vi "Calculate Voltage Difference.vi"(0 "Target Value":dbl[](array[numeric]), 2 "PowerUp?":bool, 5 "Start Value":dbl[](array[numeric])) -> (4 "Value  difference":dbl[](array[numeric]))   [LabVIEW 2024, in "devicePowerSequencerCoreLogic.lvlib"]
uses:
  devicePowerSequencerCoreLogic.lvlib
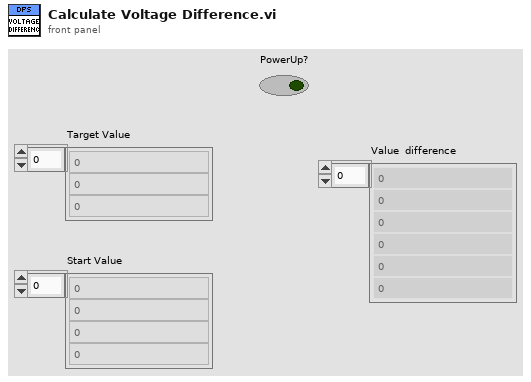
[diagram p1: front panel]
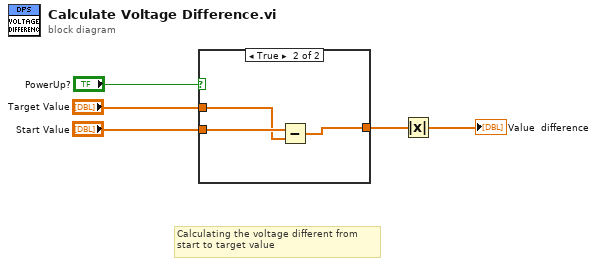
[diagram p0: block diagram]
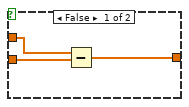
[diagram p2: hidden frame]
diagram:
  # "Calculating the voltage different from \nstart to target value"
  n1 = case shown="True" "PowerUp?" {
    tunnel: "Target Value" -> [w8 w10]
    tunnel: "Start Value" -> [w7 w11]
    tunnel: [w6 w9] -> w2
    frame False {
      n2 = Subtract(x=w8, y=w7) -> (x-y=w6:dbl[])
    }
    frame True {
      n3 = Subtract(x=w11, y=w10) -> (x-y=w9:dbl[])
    }
  }
  n4 = Absolute Value(x=w2) -> (abs(x)=→"Value  difference":dbl[])
